vi "Load.vi"(0 "User Configuration Manager":refnum<class "User Configuration Manager.lvclass">, 5 "Username":string, 7 "Password":string, 9 "Path":path, 11 "error in (no error)":errorcluster, 12 "Persistence":refnum<class "IPersist.lvclass">) -> (4 "User Configuration Manager":refnum<class "User Configuration Manager.lvclass">, 6 "Verified":bool, 8 "Verification Message":string, 15 "error out":errorcluster)   [LabVIEW 2019, in "User Configuration Manager.lvlib" / "User Configuration Manager.lvclass"]
doc: "Loads the configuration manager."
uses:
  <vilib>/gpm_packages/@cs/user-manager/Source/User Configuration Manager/User Configuration Manager.lvclass
  <vilib>/gpm_packages/@cs/persistence/source/IPersist/IPersist.lvclass
  <vilib>/gpm_packages/@cs/linked-list/Source/Linked List/Linked List/Linked List.lvclass
  C:/Program Files/National Instruments/LabVIEW 2019/vi.lib/gpm_packages/@cs/linked-list/Source/Linked List/ILinkedList/ILinked List.lvclass
  <vilib>/gpm_packages/@cs/user-manager/Source/User Configuration Manager/User Configuration Manager.lvclass/User Configuration Manager.ctl
  <vilib>/gpm_packages/@cs/user-manager/Source/User Configuration Manager/Accessors/Write Linked List ID.vi
  <vilib>/gpm_packages/@cs/user-manager/Source/User Configuration Manager/Accessors/Write Linked List Ref .vi
  <vilib>/gpm_packages/@cs/linked-list/Source/Linked List/Linked List Ref/Linked List Ref.lvclass
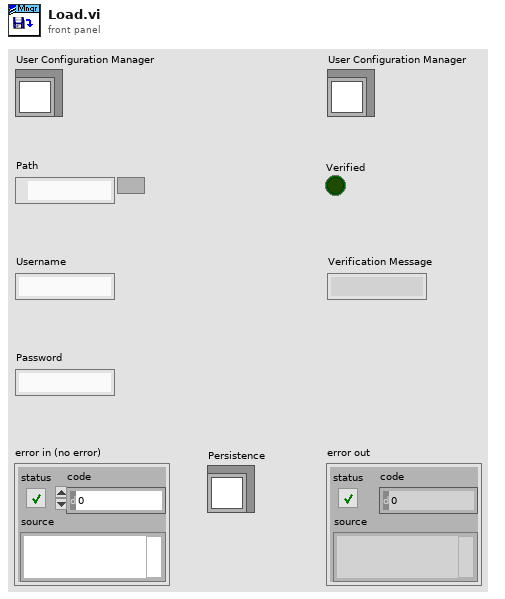
[diagram p1: front panel]
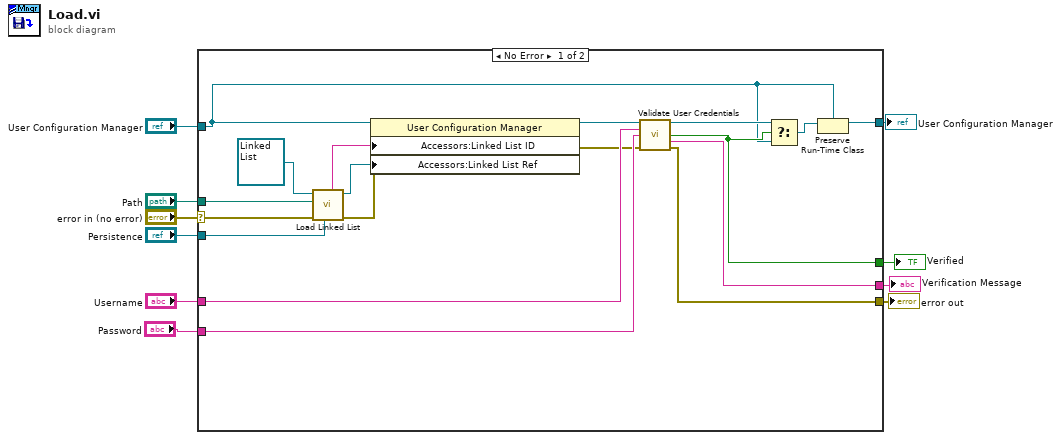
[diagram p0: block diagram]
diagram:
  n1 = case shown="No Error" "error in (no error)" {
    selector: "error in (no error)" -> [w23 w29]
    tunnel: "User Configuration Manager" -> [w11 w30]
    tunnel: "Path" -> [w24 _]
    tunnel: "Persistence" -> [w22 _]
    tunnel: "Username" -> [w19 _]
    tunnel: [w12 w30] -> w5
    tunnel: [w16 w29] -> w4
    tunnel: "Password" -> [w18 _]
    tunnel: [w20 _] -> w2
    tunnel: [w15 _] -> w1
    frame No Error {
      n2 = call <vilib>:"Load Linked List.vi"("Persistence"=w22, "error in (no error)"=w23, "File Path"=w24, "Linked List"=refnum<class "Linked List.lvclass"> refnum ("Linked Lists.lvlib:Linked List.lvclass")) -> ("error out"=w25:errorcluster, "Linked List Ref out"=w27:refnum<data-value>, "Linked List ID out"=w26:string)  [unwired: 5 in]
      n3 = property class="User Configuration Manager"(reference=w11, error in=w25, "Accessors:Linked List ID"=w26, "Accessors:Linked List Ref "=w27) -> (reference out=w21:refnum<class "User Configuration Manager.lvclass">, error out=w17:errorcluster)
      n4 = call-dynamic "Validate User Credentials.vi"("User Configuration Manager in"=w21, "Username"=w19, "Password"=w18, "error in (no error)"=w17) -> ("User Configuration Manager out"=w13:refnum<class "User Configuration Manager.lvclass">, "Verified"=w15:bool, "Verification Message"=w20:string, "error out"=w16:errorcluster)  [unwired: 7 in, 1 out]
      n5 = Select(t=w13, s=w15, f=w11) -> (s? t:f=w14:refnum<class "User Configuration Manager.lvclass">)
      n6 = Preserve Run-Time Class(object in=w14, 2:w11) -> (object out=w12:refnum<class "User Configuration Manager.lvclass">)  [unwired: 1 in, 1 out]
    }
    frame Error {
    }
  }
  "User Configuration Manager" <- w5
  "error out" <- w4
  "Verification Message" <- w2
  "Verified" <- w1
